vi "OpenSink.vi"(8 "error in (no error)":errorcluster, 11 "FileAppender in":refnum<class "FileAppender.lvclass">) -> (0 "error out":errorcluster, 3 "FileAppender out":refnum<class "FileAppender.lvclass">)   [LabVIEW 2026, in "Lumberjack.lvlib" / "FileAppender.lvclass"]
doc: "Open this appender's sink resource. Called once on actor entry (from Actor Core) before any Write. Abstract: each concrete appender opens its own sink (file, console, relay target). DD, must override."
uses:
  FileAppender.lvclass
  C:/Users/dallis/OneDrive - Velico Medical/Documents/Personal/LabVIEW Coding Projects/Lumberjack/src/Core/Appenders/Appender.lvclass/Appender.lvclass
  FileAppender.lvclass/FileAppender.ctl
  Lumberjack.lvlib
  Appender.lvclass/Appender.lvclass
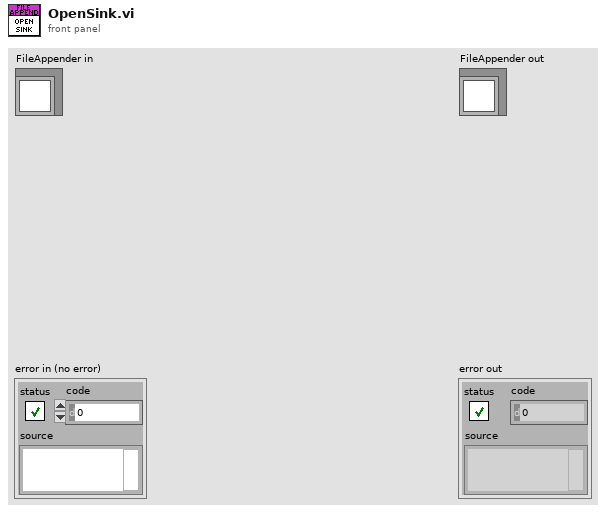
[diagram p1: front panel]
types:
  T1 = typedef "Lumberjack.lvlib/AppenderConfig.ctl" = cluster{"id":string, "threshold":T2, "filter":T3, "queueBound":i32, "dropPolicy":T5, "useUTC":bool}
  T2 = typedef "Lumberjack.lvlib/Severity.ctl" = enum16{"OFF", "FATAL", "ERROR", "WARN", "INFO", "DEBUG", "TRACE", "ALL"}
  T3 = typedef "Lumberjack.lvlib/Filter.ctl" = cluster{"mode":T4, "levelMin":T2, "levelMax":T2, "tagPrefix":string}
  T4 = typedef "Lumberjack.lvlib/FilterMode.ctl" = enum16{"Mirror", "Routed"}
  T5 = typedef "Lumberjack.lvlib/DropPolicy.ctl" = enum16{"DropOldest", "DropNewest", "LevelAware"}
  T6 = typedef "Lumberjack.lvlib/FileConfig.ctl" = cluster{"rootFolder":path, "maxFileSize":i64, "maxFileCount":i32, "baseName":string, "extension":string, "delimiter":string, "calendarFolderTree":bool}
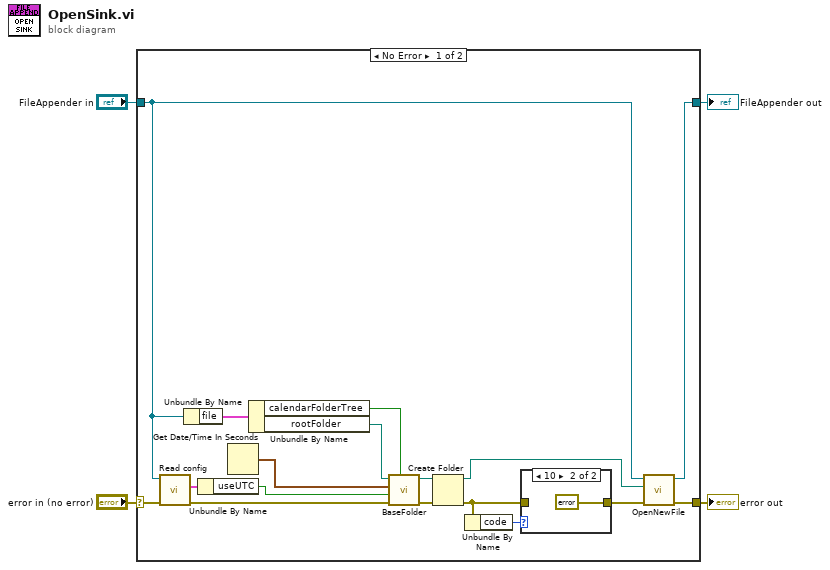
[diagram p0: block diagram]
diagram:
  n1 = case shown="No Error" "error in (no error)" {
    selector: "error in (no error)" -> [w21 w25]
    tunnel: [w12 w25] -> w4
    tunnel: [w5 w24] -> w3
    tunnel: "FileAppender in" -> [w11 w24]
    frame No Error {
      n2 = call "Read config.vi"("error in (no error)"=w21, "Appender in"=w11) -> ("error out"=w19:errorcluster, "AppenderConfig"=w18:T1)  [unwired: 7 in, 1 out]
      n3 = Unbundle By Name(w11) -> ("file"=w20:T6)
      n4 = Unbundle By Name(w18) -> ("useUTC"=w17:bool)
      n5 = Get Date/Time In Seconds() -> (seconds since 1Jan1904=w16:timestamp)
      n6 = Unbundle By Name(w20) -> ("calendarFolderTree"=w15:bool, "rootFolder"=w8:path)
      n7 = call "BaseFolder.vi"("calendarFolderTree"=w15, "error in (no error)"=w19, "useUTC"=w17, "Timestamp"=w16, "RootFolder"=w8) -> ("error out"=w13:errorcluster, "Folder"=w14:path)  [unwired: 5 in]
      n8 = Create Folder(path (use dialog)=w14, error in=w13) -> (created path=w7:path, error out=w9:errorcluster)  [unwired: 1 in, 1 out]
      n9 = Unbundle By Name(w9) -> ("code"=w10:i32)
      n10 = case shown="10" w10 {
        tunnel: w9 -> [w22 _]
        tunnel: [w22 errorcluster {"status"=FALSE, "code"=0, "source"=""} ("error out")] -> w6
        frame Default {
        }
        frame 10 {
        }
      }
      n11 = call "OpenNewFile.vi"("error in (no error)"=w6, "targetFolder"=w7, "FileAppender in"=w11) -> ("error out"=w12:errorcluster, "FileAppender out"=w5:refnum<class "FileAppender.lvclass">)  [unwired: 7 in]
    }
    frame Error {
    }
  }
  "error out" <- w4
  "FileAppender out" <- w3
